vi "Coord window-Cleanup.vi"(11 "Coordinate list window refs":T1) -> ()   [LabVIEW 2017]
uses:
  Typedefs/Coordinate list window refs.ctl
  Globals/Coord window-Globals.vi
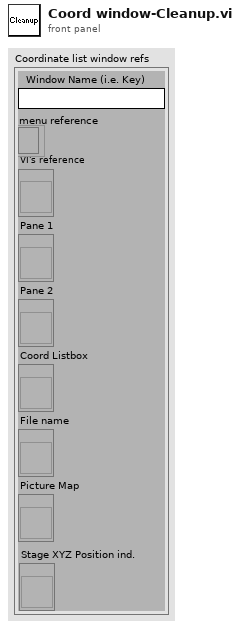
[diagram p1: front panel]
types:
  T1 = typedef "Coordinate list window refs.ctl" = cluster{"Window Name (i.e. Key)":string, "menu reference":refnum<k9>, "VI's reference":refnum<vi>, "Pane 1":refnum<vi>, "Pane 2":refnum<vi>, "Coord Listbox":refnum<vi>, "File name":refnum<vi>, "Picture Map":refnum<vi>, "Stage XYZ Position ind.":refnum<vi>}
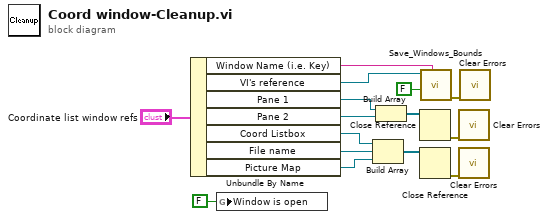
[diagram p0: block diagram]
diagram:
  n1 = Unbundle By Name("Coordinate list window refs") -> ("Window Name (i.e. Key)"=w4:string, "VI's reference"=w3:refnum<vi>, "Pane 1"=w6:refnum<vi>, "Pane 2"=w7:refnum<vi>, "Coord Listbox"=w11:refnum<vi>, "File name"=w10:refnum<vi>, "Picture Map"=w9:refnum<vi>)
  n2 = global write "Coord window-Globals.vi" "Window is open"(FALSE ("Window is open")) -> ()
  n3 = Build Array(w11, w10, w9) -> (w8:refnum<vi>[])
  n4 = Build Array(w6, w7) -> (w5:refnum<vi>[])
  n5 = Close Reference(reference=w5) -> (error out=w13:errorcluster)  [unwired: 1 in]
  n6 = Close Reference(reference=w8) -> (error out=w12:errorcluster)  [unwired: 1 in]
  n7 = call "Save_Windows_Bounds.vi"("Window Name (i.e. Key)"=w4, "Front Panel Window:Open"=FALSE, "Window VI's Ref"=w3) -> ("Error out (pass-through)"=w2:errorcluster)  [unwired: 8 in]
  n8 = call <vilib>:"Clear Errors.vi"("error in (no error)"=w13) -> ()  [unwired: 5 in, 2 out]
  n9 = call <vilib>:"Clear Errors.vi"("error in (no error)"=w12) -> ()  [unwired: 5 in, 2 out]
  n10 = call <vilib>:"Clear Errors.vi"("error in (no error)"=w2) -> ()  [unwired: 5 in, 2 out]
